vi "SLL DE DO LV2 Global Wrapper.vi"(4 "Wait for Response?":bool, 5 "Timeout (Sec)":dbl=5.0, 6 "DO value Array":bool[](array[boolean]), 7 "DO Option":T2, 8 "error in (no error)":errorcluster, 9 "DO value":bool, 10 "DO Channel Name Array":T1[](array[typedef]), 11 "DO Channel Name":T1) -> (0 "error out":errorcluster, 1 "Digital Output Array Value":bool[](array[boolean]), 2 "Digital Output Line Value":bool, 3 "Done?":bool)   [LabVIEW 2013]
uses:
  Controls/SLL DE DO Global Options.ctl
  Controls/SLL DE List of Digital Outputs.ctl
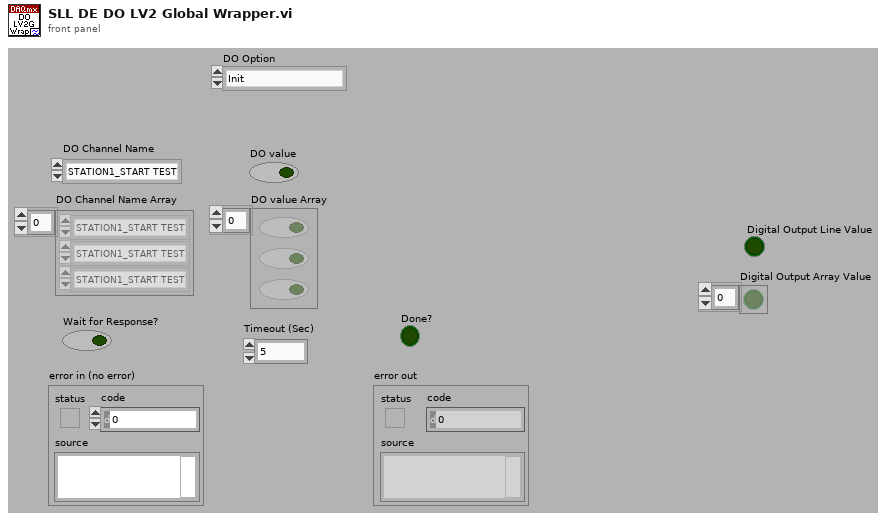
[diagram p1: front panel]
types:
  T1 = typedef "SLL DE List of Digital Outputs.ctl" = enum16{"STATION1_START TEST", "STATION1_STOP TEST", "STATION1_LIGHT1", "STATION1_LIGHT2", "STATION1_LIGHT3", "STATION1_SELECT_TEST", "STATION2_START TEST", "STATION2_STOP TEST", "STATION2_LIGHT1", "STATION2_LIGHT2", "STATION2_LIGHT3", "STATION2_SELECT_TEST", "STATION3_START TEST", "STATION3_STOP TEST", "STATION3_LIGHT1", "STATION3_LIGHT2", "STATION3_LIGHT3", "STATION3_SELECT_TEST", "STATION4_START TEST", "STATION4_STOP TEST", "STATION4_LIGHT1", "STATION4_LIGHT2", "STATION4_LIGHT3", "STATION4_SELECT_TEST"}
  T2 = typedef "SLL DE DO Global Options.ctl" = enum16{"Init", "Write Line", "Write Array", "Write Full Status", "Read Line", "Read Array", "Read Full Status", "Restart DO", "Send to Safe Mode", "Stop DO"}
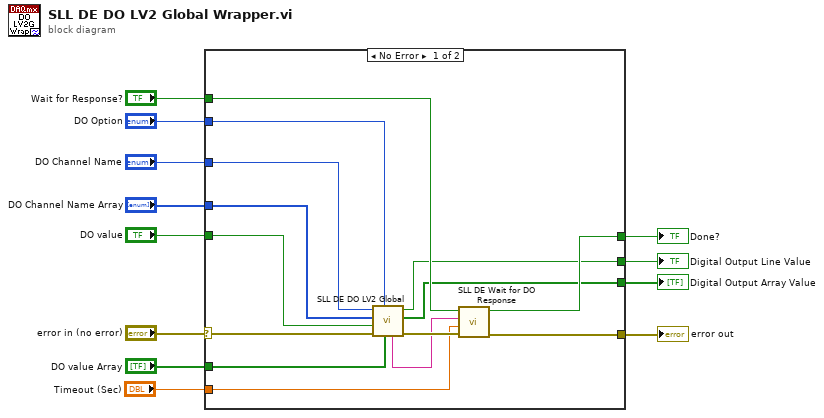
[diagram p0: block diagram]
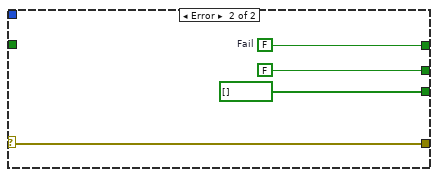
[diagram p2: hidden frame]
diagram:
  n1 = case shown="No Error" "error in (no error)" {
    selector: "error in (no error)" -> [w16 w30]
    tunnel: [w25 w30] -> w11
    tunnel: "DO Option" -> [w24 _]
    tunnel: "DO Channel Name" -> [w23 _]
    tunnel: "DO Channel Name Array" -> [w22 _]
    tunnel: "DO value" -> [w21 _]
    tunnel: "DO value Array" -> [w20 _]
    tunnel: "Wait for Response?" -> [w18 _]
    tunnel: [w17 w29] -> w4
    tunnel: [w15 FALSE] -> w3
    tunnel: [w14 bool[] [] ("Analog Output Array Value")] -> w2
    tunnel: "Timeout (Sec)" -> [w13 _]
    frame No Error {
      n2 = call "SLL DE DO LV2 Global.vi"("DO State Array"=w20, "DO Option"=w24, "Error In"=w16, "DO State"=w21, "DO Channel Name Array"=w22, "DO Channel Name"=w23) -> ("error out"=w26:errorcluster, "Digital Array Status"=w14:bool[], "Digital Line Status"=w15:bool, "Element Wrote"=w19:string)  [unwired: 2 in]
      n3 = call "SLL DE Wait for DO Response.vi"("Error In"=w26, "Timeout (Sec)"=w13, "Executed For?"=w19, "Check Response?"=w18) -> ("error out"=w25:errorcluster, "Done?"=w17:bool)  [unwired: 6 in]
    }
    frame Error {
      w29 = FALSE  # Fail
    }
  }
  "error out" <- w11
  "Done?" <- w4
  "Digital Output Line Value" <- w3
  "Digital Output Array Value" <- w2
